vi "get FPGA resources reserved by this node.vi"(8 "error in (no error)":errorcluster, 11 "Node Ptr":T1 format="%.0x") -> (0 "error out":errorcluster, 2 "reserved items":cluster{"fpga cd":T1, "resource":T2}[](array[cluster]) {"fpga cd" format="%.0x"}, 3 "Item Ref out":T1 format="%.0x")   [LabVIEW 2016, in "FPGA RM System Definition API.lvlib"]
doc: "returns all items in the SysDef reserved by this node"
uses:
  FPGA RM System Definition API.lvlib
  <vilib>/NI Veristand/Custom Device API/Custom Device Item Ref.ctl
  fpga resource.ctl
  Channel Type.ctl
  <vilib>/NI VeriStand/Custom Device API/Custom Device API.lvlib
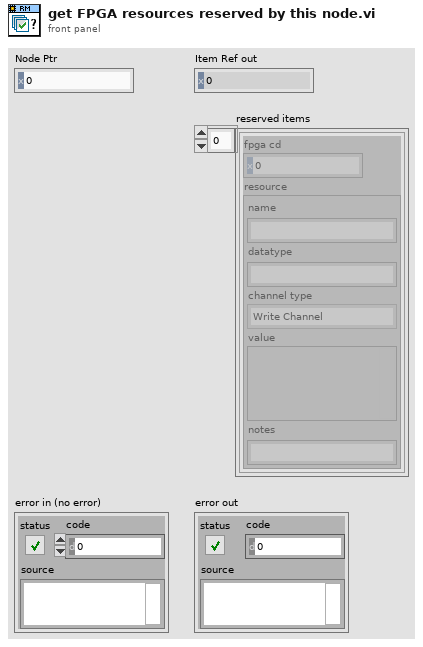
[diagram p1: front panel]
types:
  T1 = typedef "Custom Device API.lvlib/Custom Device Item Ref.ctl" = u64
  T2 = typedef "FPGA RM System Definition API.lvlib/fpga resource.ctl" = cluster{"name":string, "datatype":string, "channel type":T3, "value":variant, "notes":string}
  T3 = typedef "FPGA RM System Definition API.lvlib/Channel Type.ctl" = enum16{"Write Channel", "Read Channel", "Write Waveform", "Read Waveform"}
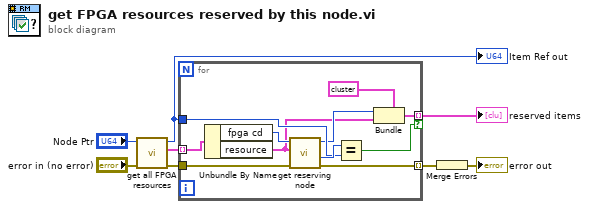
[diagram p0: block diagram]
diagram:
  n1 = call "get all FPGA resources.vi"("error in (no error)"="error in (no error)", "Item Ref in"="Node Ptr") -> ("error out"=w5:errorcluster, "fpga resources"=w3:cluster{"fpga cd":T1, "resource":T2}[], "Item Ref out"=w8:T1)  [unwired: 7 in]
  "Item Ref out" <- w8
  n2 = for {
    tunnel: w3 -> [w19] mode=indexing
    tunnel: w8 -> [w16]
    tunnel: [w10] -> w1 mode=indexing if=w15
    tunnel: w5 -> [w14]
    tunnel: [w13] -> w6 mode=indexing
    n3 = Unbundle By Name(w19) -> ("fpga cd"=w18:T1, "resource"=w11:T2)
    n4 = call "get reserving node.vi"("error in (no error)"=w14, "FPGA Resource"=w11, "Item Ref in"=w18) -> ("error out"=w13:errorcluster, "Dependent Node Ref"=w17:T1, "Item Ref out"=w12:T1)  [unwired: 5 in, 1 out]
    n5 = Equal?(x=w17, y=w16) -> (x = y?=w15:bool)
    n6 = Bundle(cluster=cluster{"fpga cd":T1, "resource":T2} {"fpga cd"=0, "resource"={"name"="", "datatype"="", "channel type"=enum."Write Channel", "value"=variant, "notes"=""}}, "fpga cd"=w12, "resource"=w11) -> (w10:cluster{"fpga cd":T1, "resource":T2})
  }
  "reserved items" <- w1
  n7 = Merge Errors(w6) -> (→"error out":errorcluster)
